vi "Configure Dispenser.vi"(7 "Config Folder":path, 8 "error in (no error)":errorcluster, 11 "WorkTable Class in":refnum<class "WorkTable Class.lvclass">) -> (0 "error out":errorcluster, 3 "WorkTable Class out":refnum<class "WorkTable Class.lvclass">)   [LabVIEW 2011, in "WorkTable Class.lvclass"]
uses:
  WorkTable Class.lvclass
  Type Definitions/Worktable_Dispenser.ctl
  <vilib>/Utility/config.llb/Read Key (String).vi
  <vilib>/Utility/config.llb/NI_LVConfig.lvlib
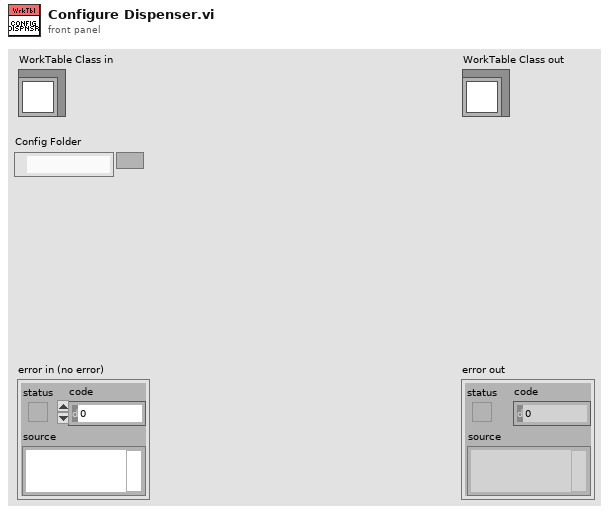
[diagram p1: front panel]
types:
  T1 = typedef "Worktable_Dispenser.ctl" = cluster{"Hardware Path":string, "Enabled":bool}
  T2 = typedef "NI_LVConfig.lvlib/Config Data RefNum.ctl" = refnum<k1>
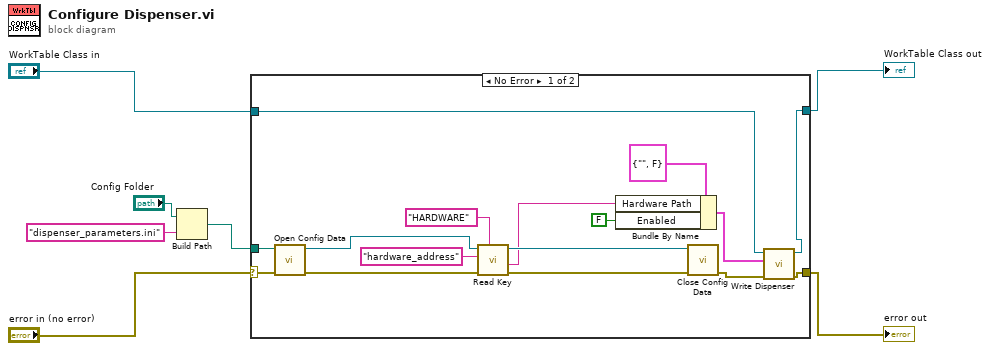
[diagram p0: block diagram]
diagram:
  n1 = Build Path(base path="Config Folder", name or relative path="dispenser_parameters.ini") -> (appended path=w5:path)
  n2 = case shown="No Error" "error in (no error)" {
    selector: "error in (no error)" -> [w22 w25]
    tunnel: [w12 w25] -> w2
    tunnel: [w15 w24] -> w1
    tunnel: "WorkTable Class in" -> [w14 w24]
    tunnel: w5 -> [w23 _]
    frame No Error {
      n3 = call <vilib>:"Open Config Data.vi"("error in (no error)"=w22, "configuration file path"=w23) -> ("error out"=w17:errorcluster, "refnum"=w19:T2)  [unwired: 7 in, 1 out]
      n4 = call-poly <vilib>:"Read Key.vi"("section"="HARDWARE", "error in (no error)"=w17, "key"="hardware_address" ("format string"), "refnum"=w19) -> ("error out"=w20:errorcluster, "value"=w9:string, "refnum out"=w21:T2)  [unwired: 4 in, 1 out]
      n5 = Bundle By Name(cluster=T1 {"Hardware Path"="", "Enabled"=FALSE} ("Dispenser"), "Hardware Path"=w9, "Enabled"=FALSE) -> (w10:T1)
      n6 = call <vilib>:"Close Config Data.vi"("error in (no error)"=w20, "refnum"=w21) -> ("error out"=w13:errorcluster)  [unwired: 8 in, 1 out]
      n7 = call-dynamic "Write Dispenser.vi"("error in (no error)"=w13, "Dispenser"=w10, "WorkTable Class in"=w14) -> ("error out"=w12:errorcluster, "WorkTable Class out"=w15:refnum<class "WorkTable Class.lvclass">)  [unwired: 7 in]
    }
    frame Error {
    }
  }
  "error out" <- w2
  "WorkTable Class out" <- w1
